vi "ConvertLocation2HeatCamPosition.vi"(6 "Transformation matrix":dbl[][](array[numeric]), 9 "yLoc":i32, 10 "xLoc":i32, 11 "Python session":refnum<k35>) -> (2 "Heat cam Y":i32, 3 "Heat cam X":i32)   [LabVIEW 2020]
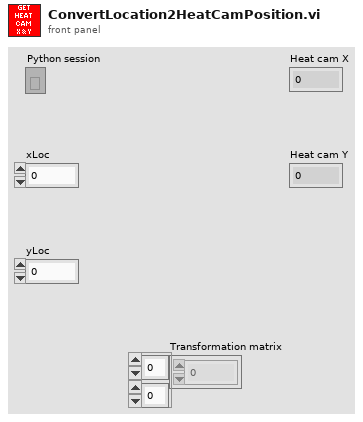
[diagram p1: front panel]
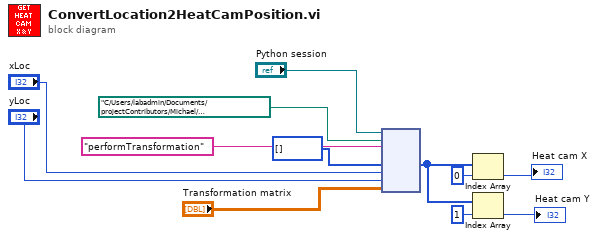
[diagram p0: block diagram]
diagram:
  n1 = node("Python session", path "C:/Users/labadmin/Documents/projectContributors/Michael/multi-larva-cl-behavior-detection/LabViewSourceCode/heatCameraPythonCode/transform.py" ("Script path"), "performTransformation" ("Function name"), i32[] [], "xLoc", "yLoc", "Transformation matrix") -> (w8:i32[])  [unwired: 4 in, 4 out]
  n2 = Index Array(array=w8, index=0) -> (element=→"Heat cam X":i32)
  n3 = Index Array(array=w8, index=1) -> (element=→"Heat cam Y":i32)
